vi "util.error.create.vi"(11 "Ring":T1 items=["[5000] Missing Function Arguments"=5000, "[5001] Incorrect Function Arguments"=5001, "[5010] Not Found"=5010, "[5050] Empty Varient Name"=5050]) -> (0 "error out":errorcluster, 3 "call chain":string[](array[string]))   [LabVIEW 2024]
uses:
  controls/typeEngErrorCodes.ctl
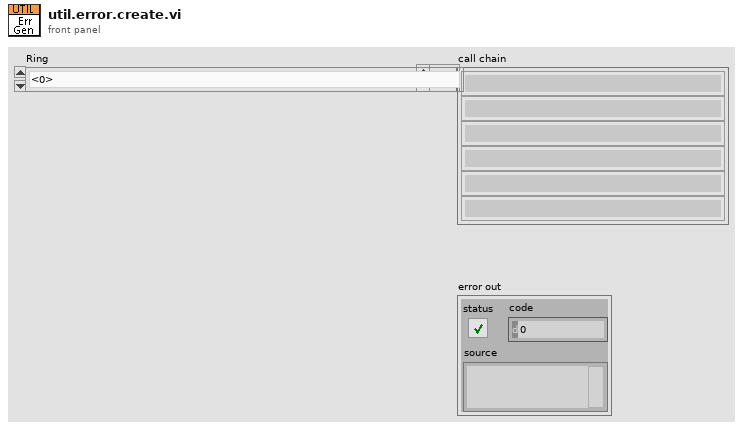
[diagram p1: front panel]
types:
  T1 = typedef "typeEngErrorCodes.ctl" = u16
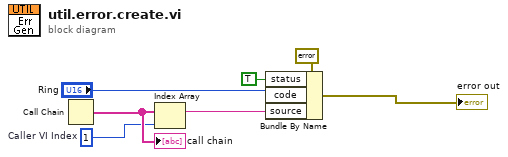
[diagram p0: block diagram]
diagram:
  w1 = 1  # Caller VI Index
  n1 = Call Chain() -> (call chain=w3:string[])
  "call chain" <- w3
  n2 = Index Array(array=w3, index=w1) -> (element=w4:string)
  n3 = Bundle By Name(cluster=errorcluster {"status"=FALSE, "code"=0, "source"=""} ("error out"), "status"=TRUE, "code"="Ring", "source"=w4) -> (→"error out":errorcluster)
